vi "9263_9264_9269 4Ch Analog Output.vi"(2 "Packets":u64[](array[numeric])=[0, 0], 4 "9263/4/9 I/O":T1={"AO0"="NI 9263/AO0", "AO1"="NI 9263/AO1", "AO2"="NI 9263/AO2", "AO3"="NI 9263/AO3"}) -> ()   [LabVIEW 2010]
uses:
  <vilib>/eio/EIONode/EIONode.xnode
  <vilib>/rvi/eio/nirviEIOImplementation/nirviEIOImplementation.xnode
  <vilib>/rvi/eio/common/nirviEmuClasses.ctl
  <vilib>/rvi/eio/common/nirviEmuTemplateMethod_noerrors.vi
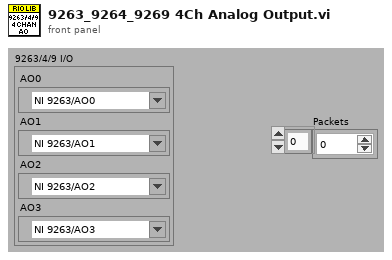
[diagram p1: front panel]
types:
  T1 = cluster{"AO0":refnum<k21>, "AO1":refnum<k21>, "AO2":refnum<k21>, "AO3":refnum<k21>}
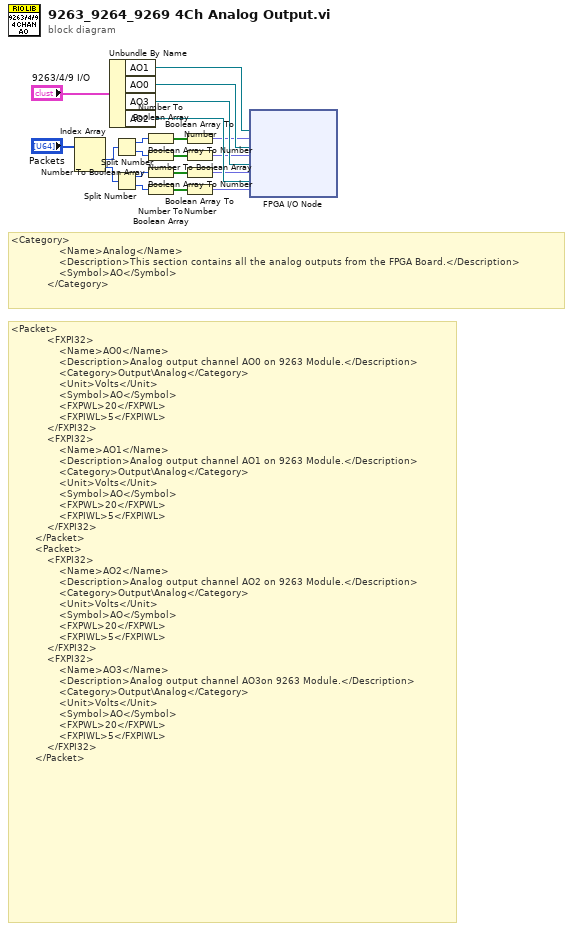
[diagram p0: block diagram]
diagram:
  # "<Category>\n                <Name>Analog</Name>\n                <Description>This section contains all the analog outputs from the FPGA Board.</Description>\n                <Symbol>AO</Symbol>\n            </Category>"
  # "<Packet>\n            <FXPI32>\n                <Name>AO0</Name>\n                <Description>Analog output channel AO0 on 9263 Module.</Description>\n                <Category>Output\\Analog</Category>\n                <Unit>Volts</Unit>\n                <Symbol>AO</Symbol>\n                <FXPWL>20</FXPWL>\n                <FXPIWL>5</FXPIWL>\n            </FXPI32>\n            <FXPI32>\n                <Name>AO1</Name>\n                <Description>Analog output channel AO1 on 9263 Module.</Description>\n                <Category>Output\\Analog</Category>\n                <Unit>Volts</Unit>\n                <Symbol>AO</Symbol>\n                <FXPWL>20</FXPWL>\n                <FXPIWL>5</FXPIWL>\n            </FXPI32>\n        </Packet>\n        <Packet>\n            <FXPI32>\n                <Name>AO2</Name>\n                <Description>Analog output channel AO2 on 9263 Module.</Description>\n                <Category>Output\\Analog</Category>\n                <Unit>Volts</Unit>\n                <Symbol>AO</Symbol>\n                <FXPWL>20</FXPWL>\n                <FXPIWL>5</FXPIWL>\n            </FXPI32>\n            <FXPI32>\n                <Name>AO3</Name>\n                <Description>Analog output channel AO3on 9263 Module.</Description>\n                <Category>Output\\Analog</Category>\n                <Unit>Volts</Unit>\n                <Symbol>AO</Symbol>\n                <FXPWL>20</FXPWL>\n                <FXPIWL>5</FXPIWL>\n            </FXPI32>\n        </Packet>"
  n1 = Index Array(array="Packets") -> (element #1=w2:u64, element #2=w3:u64)  [unwired: 2 in]
  n2 = Unbundle By Name("9263/4/9 I/O") -> ("AO1"=w19:refnum<k21>, "AO0"=w20:refnum<k21>, "AO3"=w18:refnum<k21>, "AO2"=w17:refnum<k21>)
  n3 = Split Number(x=w2) -> (hi(x)=w4:u32, lo(x)=w5:u32)
  n4 = Split Number(x=w3) -> (hi(x)=w6:u32, lo(x)=w7:u32)
  n5 = Number To Boolean Array(number=w4) -> (Boolean array=w9:bool[])
  n6 = Number To Boolean Array(number=w5) -> (Boolean array=w11:bool[])
  n7 = Number To Boolean Array(number=w6) -> (Boolean array=w12:bool[])
  n8 = Number To Boolean Array(number=w7) -> (Boolean array=w14:bool[])
  n9 = Boolean Array To Number(Boolean array=w9) -> (number=w8:fxp<+/-,20,5>)
  n10 = Boolean Array To Number(Boolean array=w11) -> (number=w10:fxp<+/-,20,5>)
  n11 = Boolean Array To Number(Boolean array=w12) -> (number=w13:fxp<+/-,20,5>)
  n12 = Boolean Array To Number(Boolean array=w14) -> (number=w15:fxp<+/-,20,5>)
  n13 = xnode "FPGA I/O Node"("I/O Item"=w8, "I/O Item"=w10, "I/O Item"=w13, "I/O Item"=w15, "FPGA I/O In"=w19, "FPGA I/O In"=w20, "FPGA I/O In"=w18, "FPGA I/O In"=w17) -> ()  [unwired: 4 out]
